vi "AlliGator Parse Python Function Input Parameters.vi"(8 "Error In":errorcluster, 9 "Source":string, 11 "Input String":string) -> (0 "Error Out":errorcluster, 1 "Function Input Parameters":T1[](array[typedef]), 3 "Output string":string)   [LabVIEW 2021, in "AlliGator Python Plugins.lvlib"]
doc: "Looks for Python Plugin Input Paramater Section Header and Footer and returns the parameter names, types and descriptions\n\nIf the section is found, the part that follows that section is returned."
uses:
  AlliGator Python Plugins.lvlib
  AlliGator Python Function Parameter Definition.ctl
  Strings/Strings.lvlib
panel:
  # "see the AlliGator License on the block diagram (Ctrl+E or Window:Show Block Diagram)"
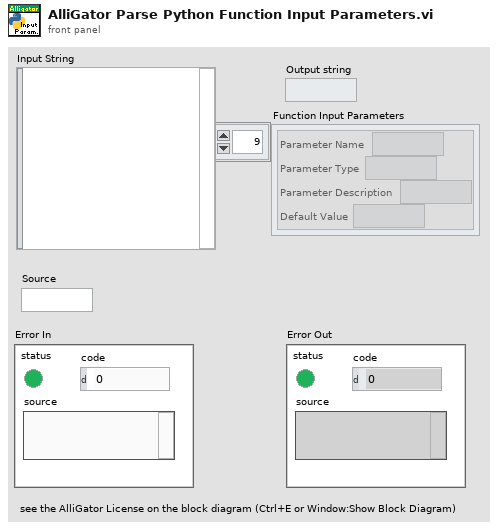
[diagram p1: front panel]
types:
  T1 = typedef "AlliGator Python Plugins.lvlib/AlliGator Python Function Parameter Definition.ctl" = cluster{"Parameter Name":string, "Parameter Type":string, "Parameter Description":string, "Default Value":string}
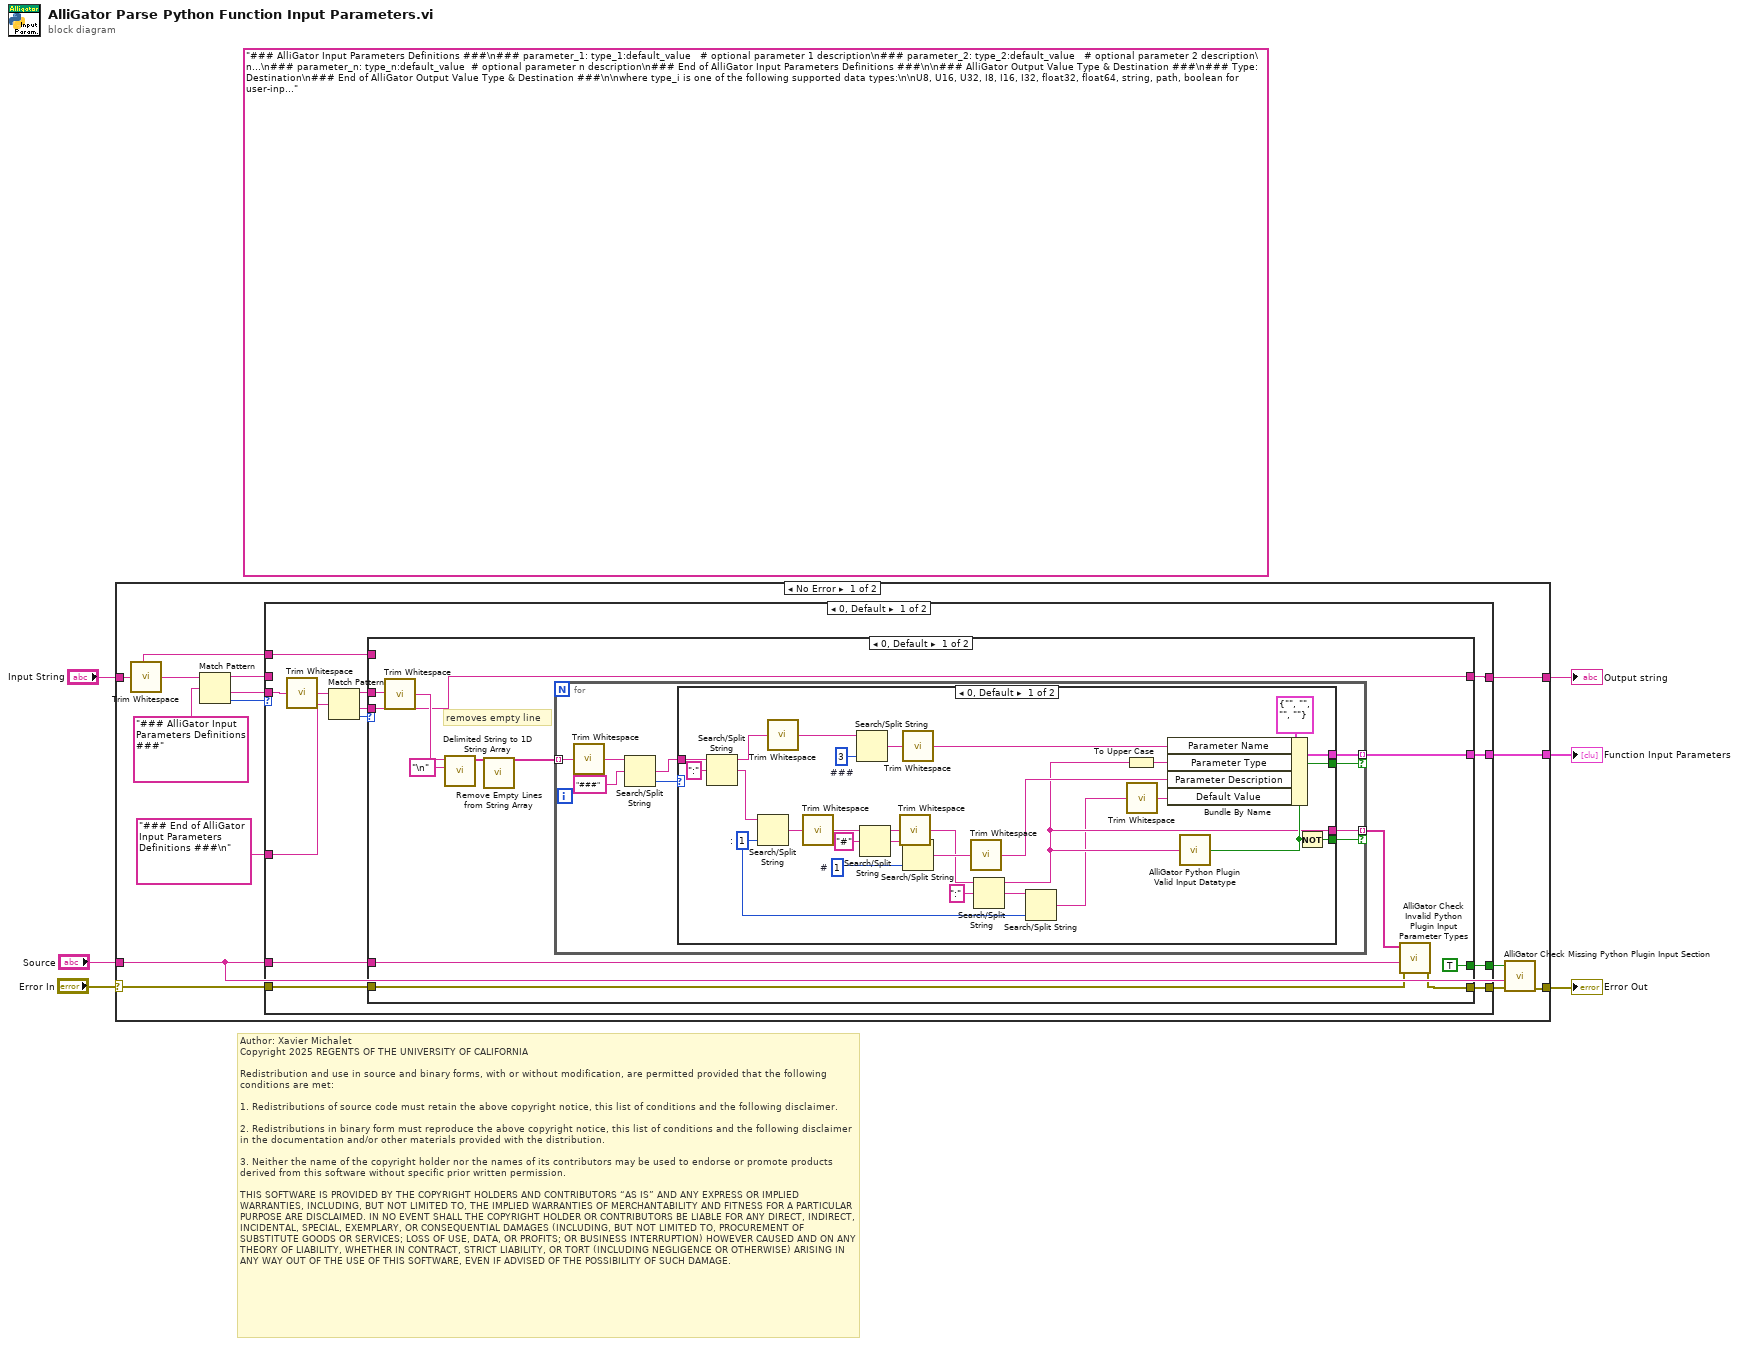
[diagram p0: block diagram]
diagram:
  (unwired) "### AlliGator Input Parameters Definitions ###\n### parameter_1: type_1:default_value   # optional parameter 1 description\n### parameter_2: type_2:default_value   # optional parameter 2 description\n...\n### parameter_n: type_n:default_value  # optional parameter n description\n### End of AlliGator Input Parameters Definitions ###\n\n### AlliGator Output Value Type & Destination ###\n### Type: Destination\n### End of AlliGator Output Value Type & Destination ###\n\nwhere type_i is one of the following supported data types:\n\nU8, U16, U32, I8, I16, I32, float32, float64, string, path, boolean for user-input parameters\nor\nAlliGator if the parameter is an internal one (in which case parameter_i needs to match the internal parameter's name exactly)\n\nThe \":default_value\" syntax is optional. If not provided, the default value is \nSupported output value_type are:\n\nplot, image, FLI dataset\n\nSupportef output destinations are:\n\ndecay graph, image sum, image max, image mask, white light image, FLI dataset"
  # "Author: Xavier Michalet\nCopyright 2025 REGENTS OF THE UNIVERSITY OF CALIFORNIA\n\nRedistribution and use in source and binary forms, with or without modification, are permitted provided that the following conditions are met:\n\n1. Redistributions of source code must retain the above copyright notice, this list of conditions and the following disclaimer.\n\n2. Redistributions in binary form must reproduce the above copyright notice, this list of conditions and the following disclaimer in the documentation and/or other materials provided with the distribution.\n\n3. Neither the name of the copyright holder nor the names of its contributors may be used to endorse or promote products derived from this software without specific prior written permission.\n\nTHIS SOFTWARE IS PROVIDED BY THE COPYRIGHT HOLDERS AND CONTRIBUTORS “AS IS” AND ANY EXPRESS OR IMPLIED WARRANTIES, INCLUDING, BUT NOT LIMITED TO, THE IMPLIED WARRANTIES OF MERCHANTABILITY AND FITNESS FOR A PARTICULAR PURPOSE ARE DISCLAIMED. IN NO EVENT SHALL THE COPYRIGHT HOLDER OR CONTRIBUTORS BE LIABLE FOR ANY DIRECT, INDIRECT, INCIDENTAL, SPECIAL, EXEMPLARY, OR CONSEQUENTIAL DAMAGES (INCLUDING, BUT NOT LIMITED TO, PROCUREMENT OF SUBSTITUTE GOODS OR SERVICES; LOSS OF USE, DATA, OR PROFITS; OR BUSINESS INTERRUPTION) HOWEVER CAUSED AND ON ANY THEORY OF LIABILITY, WHETHER IN CONTRACT, STRICT LIABILITY, OR TORT (INCLUDING NEGLIGENCE OR OTHERWISE) ARISING IN ANY WAY OUT OF THE USE OF THIS SOFTWARE, EVEN IF ADVISED OF THE POSSIBILITY OF SUCH DAMAGE."
  n1 = case shown="No Error" "Error In" {
    selector: "Error In" -> [w15 w88]
    tunnel: [w19 _] -> w6
    tunnel: "Input String" -> [w8 w87]
    tunnel: [w13 w88] -> w3
    tunnel: [w16 w87] -> w2
    tunnel: "Source" -> [w7 _]
    frame No Error {
      n2 = call <vilib>:"Trim Whitespace.vi"("string"=w8) -> ("trimmed string"=w18:string)  [unwired: 1 in]
      n3 = Match Pattern(string=w18, regular expression="### AlliGator Input Parameters Definitions ###" ("search string/char (-)")) -> (before substring=w20:string, after substring=w10:string, offset past match=w17:i32)  [unwired: 1 in, 1 out]
      n4 = case shown="0, Default" w17 {
        tunnel: w20 -> [_ _]
        tunnel: [w33 _] -> w19
        tunnel: [w26 w85] -> w16
        tunnel: "### End of AlliGator Input Parameters Definitions ###\n" ("search string/char (-)") -> [w31 _]
        tunnel: [w30 w86] -> w12
        tunnel: w15 -> [w29 w86]
        tunnel: w7 -> [w28 _]
        tunnel: [w23 _] -> w14
        tunnel: w10 -> [w25 _]
        tunnel: w8 -> [w22 w85]
        frame 0, Default {
          n5 = call <vilib>:"Trim Whitespace.vi"("string"=w25) -> ("trimmed string"=w32:string)  [unwired: 1 in]
          n6 = Match Pattern(string=w32, regular expression=w31) -> (before substring=w24:string, after substring=w21:string, offset past match=w27:i32)  [unwired: 1 in, 1 out]
          n7 = case shown="0, Default" w27 {
            tunnel: [w44 _] -> w33
            tunnel: [w39 w84] -> w30
            tunnel: w29 -> [w38 w84]
            tunnel: w28 -> [w37 _]
            tunnel: [w35 w83] -> w26
            tunnel: w24 -> [w36 _]
            tunnel: [TRUE ("Input Section Found") _] -> w23
            tunnel: w22 -> [_ w83]
            tunnel: w21 -> [w35 _]
            frame 0, Default {
              # "removes empty line"
              n8 = call <vilib>:"Trim Whitespace.vi"("string"=w36) -> ("trimmed string"=w41:string)  [unwired: 1 in]
              n9 = call <vilib>:"Delimited String to 1D String Array.vi"("delimiter"="\n", "delimited string"=w41) -> ("string array"=w43:string[])  [unwired: 9 in]
              n10 = call "Remove Empty Lines from String Array.vi"("string array in"=w43) -> ("string array out"=w42:string[])
              n11 = for {
                tunnel: w42 -> [w53] mode=indexing
                tunnel: [w54] -> w44 mode=indexing if=w52
                tunnel: [w50] -> w40 mode=indexing if=w51
                n12 = call <vilib>:"Trim Whitespace.vi"("string"=w53) -> ("trimmed string"=w49:string)  [unwired: 1 in]
                n13 = Search/Split String(string=w49, search string/char (-)="###") -> (match + rest of string=w48:string, offset of match=w46:i32)  [unwired: 1 in, 1 out]
                n14 = case shown="0, Default" w46 {
                  tunnel: [w82 _] -> w54
                  tunnel: [w78 _] -> w52
                  tunnel: [w77 _] -> w51
                  tunnel: [w60 _] -> w50
                  tunnel: w48 -> [w67 _]
                  frame 0, Default {
                    w58 = 1  # #
                    w79 = 3  # ###
                    w57 = 1  # :
                    n15 = Search/Split String(string=w67, search string/char (-)=":") -> (substring before match=w72:string, match + rest of string=w80:string)  [unwired: 1 in, 1 out]
                    n16 = Search/Split String(string=w80, offset (0)=w57) -> (match + rest of string=w75:string)  [unwired: 1 in, 2 out]
                    n17 = call <vilib>:"Trim Whitespace.vi"("string"=w72) -> ("trimmed string"=w73:string)  [unwired: 1 in]
                    n18 = call <vilib>:"Trim Whitespace.vi"("string"=w75) -> ("trimmed string"=w70:string)  [unwired: 1 in]
                    n19 = Search/Split String(string=w73, offset (0)=w79) -> (match + rest of string=w71:string)  [unwired: 1 in, 2 out]
                    n20 = Search/Split String(string=w70, search string/char (-)="#") -> (substring before match=w74:string, match + rest of string=w65:string)  [unwired: 1 in, 1 out]
                    n21 = call <vilib>:"Trim Whitespace.vi"("string"=w74) -> ("trimmed string"=w61:string)  [unwired: 1 in]
                    n22 = call <vilib>:"Trim Whitespace.vi"("string"=w71) -> ("trimmed string"=w68:string)  [unwired: 1 in]
                    n23 = Search/Split String(string=w65, offset (0)=w58) -> (match + rest of string=w64:string)  [unwired: 1 in, 2 out]
                    n24 = call <vilib>:"Trim Whitespace.vi"("string"=w64) -> ("trimmed string"=w63:string)  [unwired: 1 in]
                    n25 = Search/Split String(string=w61, search string/char (-)=":") -> (substring before match=w60:string, match + rest of string=w59:string)  [unwired: 1 in, 1 out]
                    n26 = Search/Split String(string=w59, offset (0)=w57) -> (match + rest of string=w56:string)  [unwired: 1 in, 2 out]
                    n27 = To Upper Case(1:w60) -> (0:w66:string)
                    n28 = call <vilib>:"Trim Whitespace.vi"("string"=w56) -> ("trimmed string"=w55:string)  [unwired: 1 in]
                    n29 = Bundle By Name(cluster=T1 {"Parameter Name"="", "Parameter Type"="", "Parameter Description"="", "Default Value"=""} ("Function Parameters"), "Parameter Name"=w68, "Parameter Type"=w66, "Parameter Description"=w63, "Default Value"=w55) -> (w82:T1)
                    n30 = call "AlliGator Python Plugin Valid Input Datatype.vi"("Input Datatype"=w60) -> ("Valid Datatype?"=w78:bool)  [unwired: 8 in]
                    n31 = Not(x=w78) -> (.not. x?=w77:bool)
                  }
                  frame -1 {
                  }
                }
              }
              n32 = call "AlliGator Check Invalid Python Plugin Input Parameter Types.vi"("error in (no error)"=w38, "Source"=w37, "Invalid Parameter Types"=w40) -> ("error out"=w39:errorcluster)  [unwired: 8 in]
            }
            frame -1 {
            }
          }
        }
        frame -1 {
          # "No Input Parameters section"
        }
      }
      n33 = call "AlliGator Check Missing Python Plugin Input Section.vi"("error in (no error)"=w12, "Source"=w7, "Input Section Found"=w14) -> ("error out"=w13:errorcluster)  [unwired: 8 in]
    }
    frame Error {
    }
  }
  "Function Input Parameters" <- w6
  "Error Out" <- w3
  "Output string" <- w2
